vi "Get Sender.vi"(11 "Merge Error Msg Strategy in":refnum<class "Merge Error Msg Strategy.lvclass">) -> (2 "Sender":refnum<class "Sender.lvclass">)   [LabVIEW 2021, in "Merge Error Msg Strategy.lvlib" / "Merge Error Msg Strategy.lvclass"]
uses:
  Merge Error Msg Strategy.lvclass
  Merge Error Msg Strategy.lvclass/Merge Error Msg Strategy.ctl
  jettl/Sender/Sender/Sender.lvclass
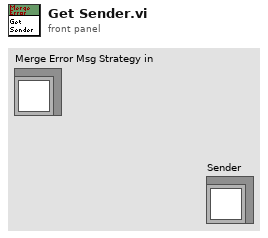
[diagram p1: front panel]
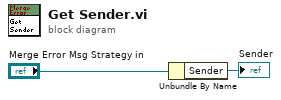
[diagram p0: block diagram]
diagram:
  n1 = Unbundle By Name("Merge Error Msg Strategy in") -> ("Sender"=→"Sender":refnum<class "Sender.lvclass">)
